vi "compare doubles.vi"(1 "base value":dbl, 4 "value to compare":dbl) -> (17 "Equal":bool)   [LabVIEW 2014, in "PTUtils.lvlib"]
uses:
  PTUtils.lvlib
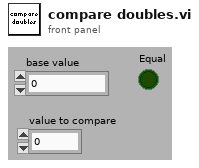
[diagram p1: front panel]
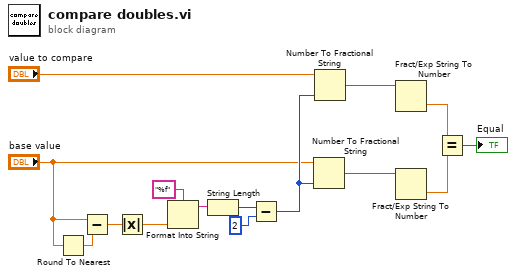
[diagram p0: block diagram]
diagram:
  n1 = Round To Nearest(number="base value") -> (nearest integer value=w15:dbl)
  n2 = Subtract(x="base value", y=w15) -> (x-y=w2:dbl)
  n3 = Absolute Value(x=w2) -> (abs(x)=w1:dbl)
  n4 = Format Into String(format string="%f", w1) -> (resulting string=w11:string)  [unwired: 2 in, 1 out]
  n5 = String Length(string=w11) -> (length=w13:i32)
  n6 = Subtract(x=w13, y=2) -> (x-y=w9:i32)
  n7 = Number To Fractional String(number="base value", precision (6)=w9) -> (F-format string=w5:string)  [unwired: 2 in]
  n8 = Number To Fractional String(number="value to compare", precision (6)=w9) -> (F-format string=w6:string)  [unwired: 2 in]
  n9 = Fract/Exp String To Number(string=w6) -> (number=w4:dbl)  [unwired: 3 in, 1 out]
  n10 = Fract/Exp String To Number(string=w5) -> (number=w3:dbl)  [unwired: 3 in, 1 out]
  n11 = Equal?(x=w4, y=w3) -> (x = y?=→"Equal":bool)
